vi "LOGIN-VI.vi"() -> (2 "Access Guaranteed?":bool)   [LabVIEW 2022 SP3]
doc: "Example of Dialog Using Events template.\n\nThis VI verifies a user login and password. The informatin for valid users is inside a table in the subvi Authenticate user.vi. The Verified? indicator will turn on if the user is valid."
panel:
  in  "Password":string
  in  "Login":string
  in  "Cancel":bool
  in  "Connect":bool
  # "This interface verifies if the \"Login\"\n& \"PWD\" are correct or not."
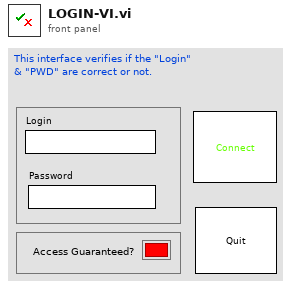
[diagram p1: front panel]
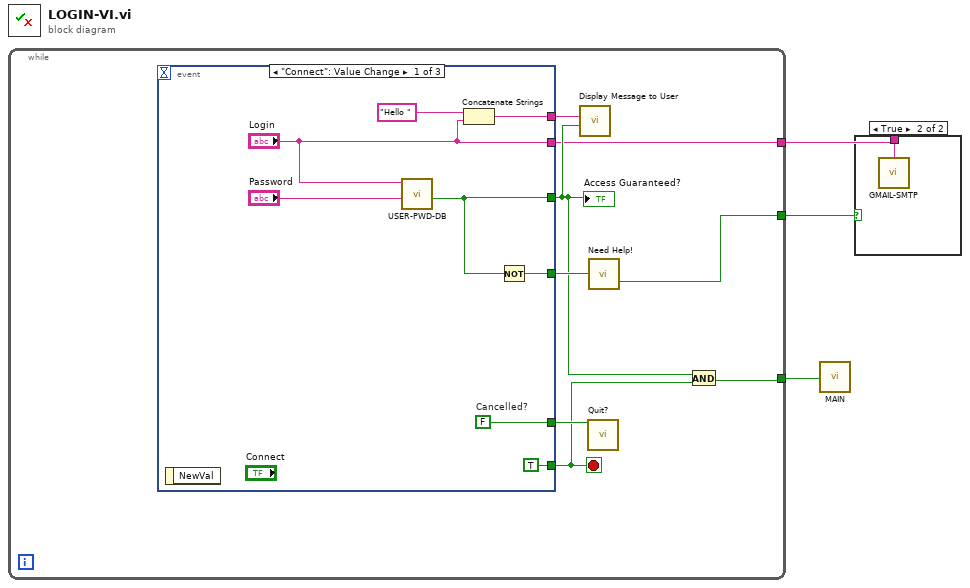
[diagram p0: block diagram]
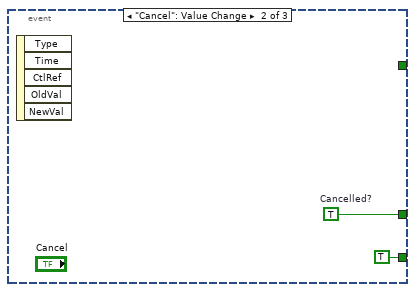
[diagram p3: hidden frame]
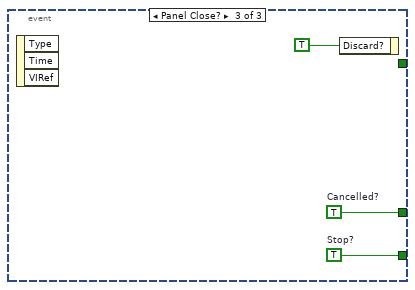
[diagram p4: hidden frame]
diagram:
  n1 = while {
    tunnel: [w6] -> w3
    tunnel: [w5] -> w2
    tunnel: [w4] -> w1
    stop <- w7 stop-if-true
    n2 = event shown="[0] \"Connect\": Value Change" {
      selector: _ -> [_ _ _]
      dyn-events: _ -> [_ _ _]
      timeout: _ -> [_ _ _]
      tunnel: [TRUE ("Stop?") TRUE ("Stop?") w23] -> w7
      tunnel: [w19 w21 w22] -> w11
      tunnel: [w14 _ _] -> w8
      tunnel: [w16 _ _] -> w10
      tunnel: [w15 _ _] -> w9
      tunnel: ["Login" _ _] -> w5
      event "Connect": Value Change {
        w19 = FALSE  # Cancelled?
        n3 = event-data() -> ()  [unwired: 1 in, 1 out]
        n4 = call "USER-PWD-DB.vi"("Password"="Password", "Login"="Login") -> ("Verified?"=w14:bool)  [unwired: 5 in]
        n5 = Concatenate Strings("Hello ", "Login") -> (w16:string)
        n6 = Not(x=w14) -> (.not. x?=w15:bool)
      }
      event "Cancel": Value Change {
        w21 = TRUE  # Cancelled?
        n7 = event-data() -> ()  [unwired: 1 in, 5 out]
      }
      event Panel Close? {
        w22 = TRUE  # Cancelled?
        w23 = TRUE  # Stop?
        n8 = event-data() -> ()  [unwired: 1 in, 3 out]
        n9 = event-data("Discard?"=TRUE) -> ()  [unwired: 1 in, 1 out]
      }
    }
    "Access Guaranteed?" <- w8
    n10 = call "Display Message to User"("Enable"=w8, "Message"=w10) -> ()  [unwired: 8 in, 2 out]
    n11 = call "Quit?"("Enable"=w11) -> ()  [unwired: 17 in, 2 out]
    n12 = call "Need Help!"("Enable"=w9) -> ("SOS"=w4:bool)  [unwired: 17 in, 1 out]
    n13 = And(x=w8, y=w7) -> (x .and. y?=w6:bool)
  }
  n14 = call "MAIN.vi"("Enable"=w3) -> ()  [unwired: 1 in]
  n15 = case shown="True" w1 {
    tunnel: w2 -> [_ w25]
    frame False {
    }
    frame True {
      n16 = call "GMAIL-SMTP.vi"("Sender's Name"=w25) -> ()  [unwired: 1 in]
    }
  }
